vi "Facade.vi"(0 "Data In":T5, 2 "Display State In":T3, 3 "Container State":T4) -> (6 "Data Out":T5, 7 "Display State Out":T3, 8 "Action":T2)   [LabVIEW 2021, in "roboRIO 10 Bank.xctl"]
uses:
  <vilib>/myRIO/Common/Instrument Driver Framework/Utilities/xctls/roboRIO 10 Bank/roboRIO 10 Bank.xctl
  <vilib>/myRIO/Common/Instrument Driver Framework/Utilities/xctls/roboRIO 10 Bank/Data.ctl
  <vilib>/_xctls/Container State.ctl
  <vilib>/myRIO/Common/Instrument Driver Framework/Utilities/xctls/roboRIO 10 Bank/State.ctl
  <vilib>/_xctls/Action.ctl
  <vilib>/_xctls/XControlSupport.lvlib
panel:
  out "Connecotr Name":string
  in  "roboRIO 10 Bank":T1
  out "Row Name 2":string caption="Port Name"
  out "Row Name 1":string caption="Port Name"
  # "Color"
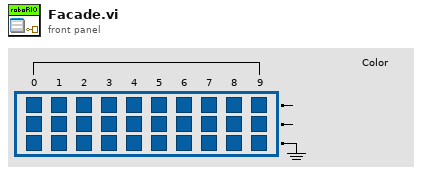
[diagram p1: front panel]
types:
  T1 = cluster{"0":bool, "1":bool, "2":bool, "3":bool, "4":bool, "5":bool, "6":bool, "7":bool, "8":bool, "9":bool, "10":bool, "11":bool, "12":bool, "13":bool, "14":bool, "15":bool, "16":bool, "17":bool, "18":bool, "19":bool, "20":bool, "21":bool, "22":bool, "23":bool, "24":bool, "25":bool, "26":bool, "27":bool, "28":bool, "29":bool}
  T2 = typedef "XControlSupport.lvlib/Action.ctl" = cluster{"Data Changed?":bool, "State Changed?":bool, "Action Name":string}
  T3 = typedef "roboRIO 10 Bank.xctl/State.ctl" = cluster{"Pin Disabled?":enum8{"Enabled", "Disabled", "Disabled and Grayed Out"}[], "Pin Name":string[], "Pin ID":string[], "Connector Name":string, "Row Name 1":string, "Row Name 2":string}
  T4 = typedef "XControlSupport.lvlib/Container State.ctl" = cluster{"Indicator?":bool, "Run Mode?":bool, " Refnum":refnum<vi>}
  T5 = typedef "roboRIO 10 Bank.xctl/Data.ctl" = bool[]
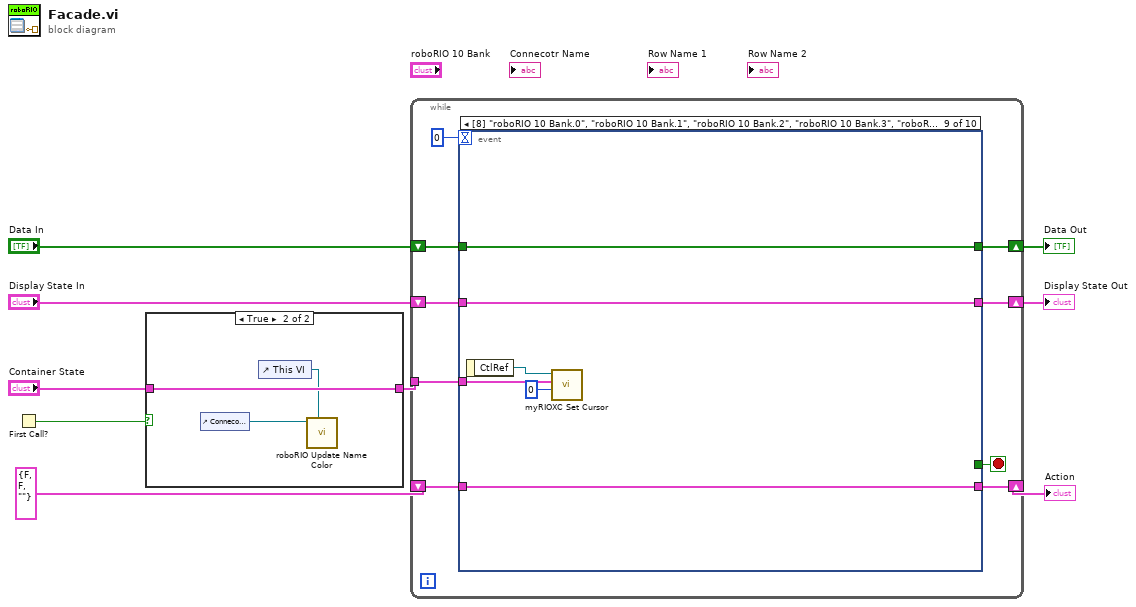
[diagram p0: block diagram]
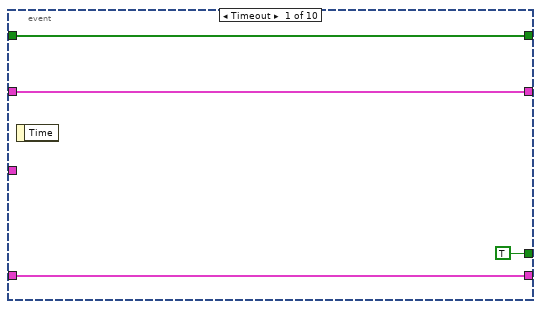
[diagram p3: hidden frame]
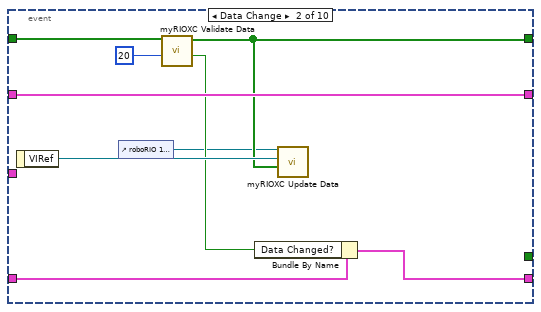
[diagram p4: hidden frame]
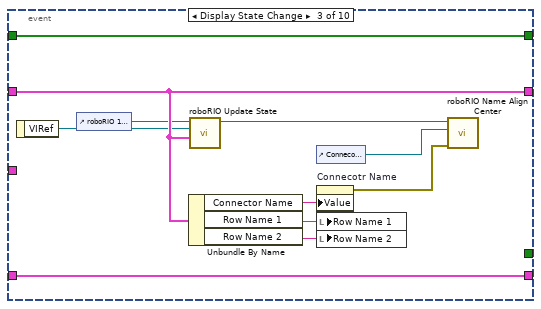
[diagram p5: hidden frame]
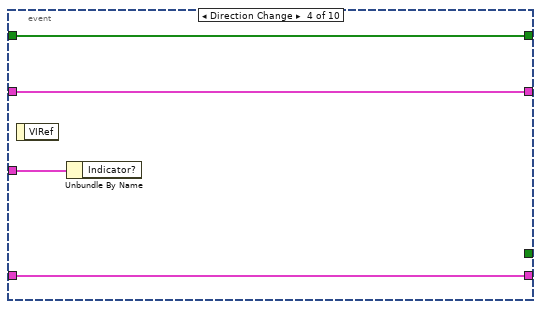
[diagram p6: hidden frame]
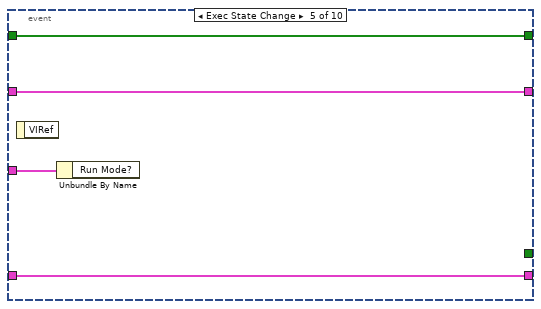
[diagram p7: hidden frame]
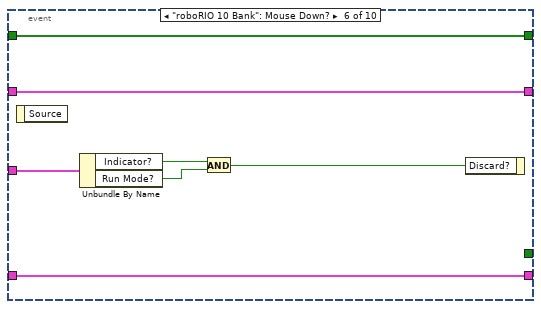
[diagram p8: hidden frame]
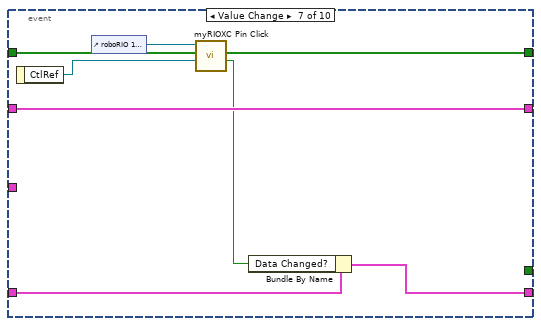
[diagram p9: hidden frame]
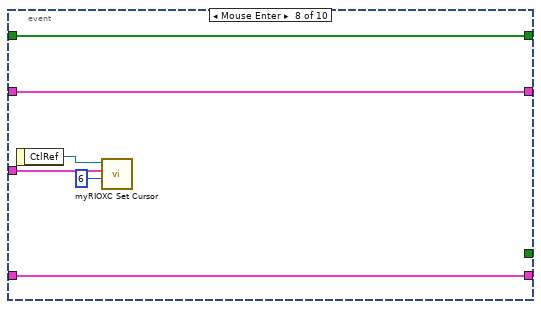
[diagram p10: hidden frame]
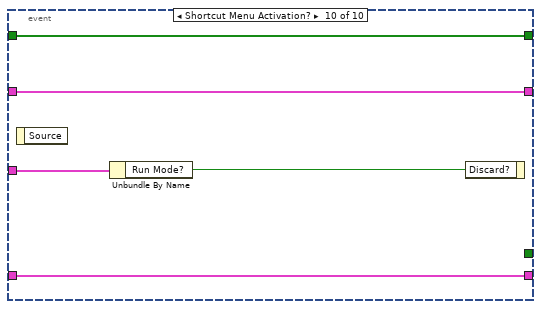
[diagram p11: hidden frame]
diagram:
  n1 = First Call?() -> (First Call?: T/F=w1:bool)
  n2 = case shown="True" w1 {
    tunnel: "Container State" -> [w10 w13]
    tunnel: [w10 w13] -> w2
    frame False {
    }
    frame True {
      n3 = control-ref of="Connecotr Name"() -> (w11:refnum<vi>)
      n4 = control-ref of="This VI"() -> (w12:refnum<vi>)
      n5 = call <vilib>:"roboRIO Update Name Color.vi"("FcdVI Ref"=w12, "Connector Name Ref"=w11) -> ()  [unwired: 9 in, 1 out]
    }
  }
  n6 = while {
    shift-right: [w21] -> w7
    shift-left: "Display State In" -> [w22]
    tunnel: w2 -> [w19]
    shift-right: [w17] -> w9
    shift-left: "Data In" -> [w18]
    shift-right: [w15] -> w5
    shift-left: T2 {"Data Changed?"=FALSE, "State Changed?"=FALSE, "Action Name"=""} ("Action") -> [w16]
    stop <- w20 stop-if-true
    n7 = event shown="[8] \"roboRIO 10 Bank.0\", \"roboRIO 10 Bank.1\", \"roboRIO 10 Bank.2\", \"roboRIO 10 Bank.3\", \"roboRIO 10 Bank.4\", \"roboRIO 10 Bank.5\", \"roboRIO 10 Bank.6\", \"roboRIO 10 Bank.7\", \"roboRIO 10 Bank.8\", \"roboRIO 10 Bank.9\", \"roboRIO 10 Bank.10\", \"roboRIO 10 Bank.11\", \"roboRIO 10 Bank.12\", \"roboRIO 10 Bank.13\", \"roboRIO 10 Bank.14\", \"roboRIO 10 Bank.15\", \"roboRIO 10 Bank.16\", \"roboRIO 10 Bank.17\", \"roboRIO 10 Bank.18\", \"roboRIO 10 Bank.19\", \"roboRIO 10 Bank.20\", \"roboRIO 10 Bank.21\", \"roboRIO 10 Bank.22\", \"roboRIO 10 Bank.23\", \"roboRIO 10 Bank.24\", \"roboRIO 10 Bank.25\", \"roboRIO 10 Bank.26\", \"roboRIO 10 Bank.27\", \"roboRIO 10 Bank.28\", \"roboRIO 10 Bank.29\": Mouse Leave" {
      selector: _ -> [_ _ _ _ _ _ _ _ _ _]
      dyn-events: _ -> [_ _ _ _ _ _ _ _ _ _]
      timeout: 0 -> [_ _ _ _ _ _ _ _ _ _]
      tunnel: w22 -> [w24 w33 w41 w48 w52 w60 w68 w74 w80 w82]
      tunnel: [w24 w33 w41 w48 w52 w60 w68 w74 w80 w82] -> w21
      tunnel: [TRUE _ _ _ _ _ _ _ _ _] -> w20
      tunnel: w19 -> [_ _ _ w49 w53 w57 _ w70 w76 w81]
      tunnel: w18 -> [w23 w32 w45 w47 w51 w59 w63 w73 w79 w85]
      tunnel: [w23 w28 w45 w47 w51 w59 w64 w73 w79 w85] -> w17
      tunnel: [w25 w34 w44 w46 w50 w58 w66 w72 w78 w84] -> w15
      tunnel: w16 -> [w25 w35 w44 w46 w50 w58 w67 w72 w78 w84]
      event Timeout {
        n8 = event-data() -> ()  [unwired: 1 in, 1 out]
      }
      event Data Change {
        n9 = event-data() -> ("VIRef"=w30:refnum<vi>)  [unwired: 1 in]
        n10 = control-ref of="roboRIO 10 Bank"() -> (w27:refnum<vi>)
        n11 = call <vilib>:"myRIOXC Validate Data.vi"("Size"=20, "Data In"=w32) -> ("Data Changed?"=w29:bool, "Data Out"=w28:bool[])  [unwired: 8 in]
        n12 = Bundle By Name(cluster=w35, "Data Changed?"=w29) -> (w34:T2)
        n13 = call <vilib>:"myRIOXC Update Data.vi"("Data In"=w28, "Facade Ref"=w30, "Connector Ref"=w27) -> ()  [unwired: 8 in, 1 out]
      }
      event Display State Change {
        n14 = event-data() -> ("VIRef"=w40:refnum<vi>)  [unwired: 1 in]
        n15 = control-ref of="roboRIO 10 Bank"() -> (w38:refnum<vi>)
        n16 = Unbundle By Name(w41) -> ("Connector Name"=w39:string, "Row Name 1"=w43:string, "Row Name 2"=w42:string)
        n17 = call <vilib>:"roboRIO Update State.vi"("Display State In"=w41, "Facade Ref"=w40, "Connector Ref"=w38) -> ()  [unwired: 8 in, 1 out]
        n18 = control-ref of="Connecotr Name"() -> (w37:refnum<vi>)
        n19 = property on="Connecotr Name" class="Str"("Value"=w39) -> (error out=w36:errorcluster)  [unwired: 2 in, 1 out]
        n20 = local write "Row Name 1"(w43) -> ()
        n21 = local write "Row Name 2"(w42) -> ()
        n22 = call <vilib>:"roboRIO Name Align Center.vi"("error in (no error)"=w36, "Target Refnum"=w37, "Ref Control"=w38) -> ()  [unwired: 8 in, 1 out]
      }
      event Direction Change {
        n23 = event-data() -> ()  [unwired: 1 in, 1 out]
        n24 = Unbundle By Name(w49) -> ()  [unwired: 1 out]
      }
      event Exec State Change {
        n25 = event-data() -> ()  [unwired: 1 in, 1 out]
        n26 = Unbundle By Name(w53) -> ()  [unwired: 1 out]
      }
      event "roboRIO 10 Bank": Mouse Down? {
        n27 = event-data() -> ()  [unwired: 1 in, 1 out]
        n28 = Unbundle By Name(w57) -> ("Indicator?"=w56:bool, "Run Mode?"=w55:bool)
        n29 = And(x=w56, y=w55) -> (x .and. y?=w54:bool)
        n30 = event-data("Discard?"=w54) -> ()  [unwired: 1 in, 1 out]
      }
      event "roboRIO 10 Bank.0", "roboRIO 10 Bank.1", "roboRIO 10 Bank.2", "roboRIO 10 Bank.3", "roboRIO 10 Bank.4", "roboRIO 10 Bank.5", "roboRIO 10 Bank.6", "roboRIO 10 Bank.7", "roboRIO 10 Bank.8", "roboRIO 10 Bank.9", "roboRIO 10 Bank.10", "roboRIO 10 Bank.11", "roboRIO 10 Bank.12", "roboRIO 10 Bank.13", "roboRIO 10 Bank.14", "roboRIO 10 Bank.15", "roboRIO 10 Bank.16", "roboRIO 10 Bank.17", "roboRIO 10 Bank.18", "roboRIO 10 Bank.19", "roboRIO 10 Bank.20", "roboRIO 10 Bank.21", "roboRIO 10 Bank.22", "roboRIO 10 Bank.23", "roboRIO 10 Bank.24", "roboRIO 10 Bank.25", "roboRIO 10 Bank.26", "roboRIO 10 Bank.27", "roboRIO 10 Bank.28", "roboRIO 10 Bank.29": Value Change {
        n31 = event-data() -> ("CtlRef"=w62:refnum<vi>)  [unwired: 1 in]
        n32 = control-ref of="roboRIO 10 Bank"() -> (w61:refnum<vi>)
        n33 = call <vilib>:"myRIOXC Pin Click.vi"("Pin Ref"=w62, "Data In"=w63, "Connector Ref"=w61) -> ("Value Change?"=w65:bool, "Data Out"=w64:bool[])  [unwired: 6 in, 1 out]
        n34 = Bundle By Name(cluster=w67, "Data Changed?"=w65) -> (w66:T2)
      }
      event "roboRIO 10 Bank.0", "roboRIO 10 Bank.1", "roboRIO 10 Bank.2", "roboRIO 10 Bank.3", "roboRIO 10 Bank.4", "roboRIO 10 Bank.5", "roboRIO 10 Bank.6", "roboRIO 10 Bank.7", "roboRIO 10 Bank.8", "roboRIO 10 Bank.9", "roboRIO 10 Bank.10", "roboRIO 10 Bank.11", "roboRIO 10 Bank.12", "roboRIO 10 Bank.13", "roboRIO 10 Bank.14", "roboRIO 10 Bank.15", "roboRIO 10 Bank.16", "roboRIO 10 Bank.17", "roboRIO 10 Bank.18", "roboRIO 10 Bank.19", "roboRIO 10 Bank.20", "roboRIO 10 Bank.21", "roboRIO 10 Bank.22", "roboRIO 10 Bank.23", "roboRIO 10 Bank.24", "roboRIO 10 Bank.25", "roboRIO 10 Bank.26", "roboRIO 10 Bank.27", "roboRIO 10 Bank.28", "roboRIO 10 Bank.29": Mouse Enter {
        n35 = event-data() -> ("CtlRef"=w69:refnum<vi>)  [unwired: 1 in]
        n36 = call <vilib>:"myRIOXC Set Cursor.vi"("Cursor"=u16 6, "Container State"=w70, "PIN Ref"=w69) -> ()  [unwired: 9 in]
      }
      event "roboRIO 10 Bank.0", "roboRIO 10 Bank.1", "roboRIO 10 Bank.2", "roboRIO 10 Bank.3", "roboRIO 10 Bank.4", "roboRIO 10 Bank.5", "roboRIO 10 Bank.6", "roboRIO 10 Bank.7", "roboRIO 10 Bank.8", "roboRIO 10 Bank.9", "roboRIO 10 Bank.10", "roboRIO 10 Bank.11", "roboRIO 10 Bank.12", "roboRIO 10 Bank.13", "roboRIO 10 Bank.14", "roboRIO 10 Bank.15", "roboRIO 10 Bank.16", "roboRIO 10 Bank.17", "roboRIO 10 Bank.18", "roboRIO 10 Bank.19", "roboRIO 10 Bank.20", "roboRIO 10 Bank.21", "roboRIO 10 Bank.22", "roboRIO 10 Bank.23", "roboRIO 10 Bank.24", "roboRIO 10 Bank.25", "roboRIO 10 Bank.26", "roboRIO 10 Bank.27", "roboRIO 10 Bank.28", "roboRIO 10 Bank.29": Mouse Leave {
        n37 = event-data() -> ("CtlRef"=w75:refnum<vi>)  [unwired: 1 in]
        n38 = call <vilib>:"myRIOXC Set Cursor.vi"("Cursor"=u16 0, "Container State"=w76, "PIN Ref"=w75) -> ()  [unwired: 9 in]
      }
      event Shortcut Menu Activation? {
        n39 = event-data() -> ()  [unwired: 1 in, 1 out]
        n40 = Unbundle By Name(w81) -> ("Run Mode?"=w83:bool)
        n41 = event-data("Discard?"=w83) -> ()  [unwired: 1 in, 1 out]
      }
    }
  }
  "Display State Out" <- w7
  "Data Out" <- w9
  "Action" <- w5
